vi "Query Protection Status.vi"(8 "error in (no error)":errorcluster, 10 "Channel (1)":string="1", 11 "VISA resource name":refnum<visa-resource-name>) -> (0 "error out":errorcluster, 1 "OCP Tripped":bool[](array[boolean]), 2 "OVP Tripped":bool[](array[boolean]), 3 "VISA resource name out":refnum<visa-resource-name>)   [LabVIEW 2020, in "Keysight E36300 Series.lvlib"]
doc: "Returns Overvoltage Protection (OVP) and Overcurrent Protection (OCP) status for a desired channel."
uses:
  Keysight E36300 Series.lvlib
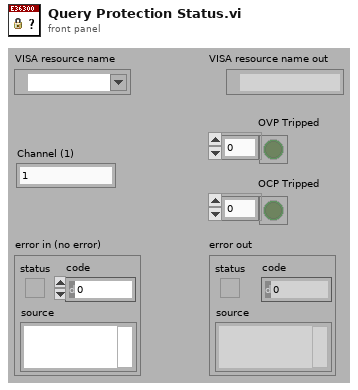
[diagram p1: front panel]
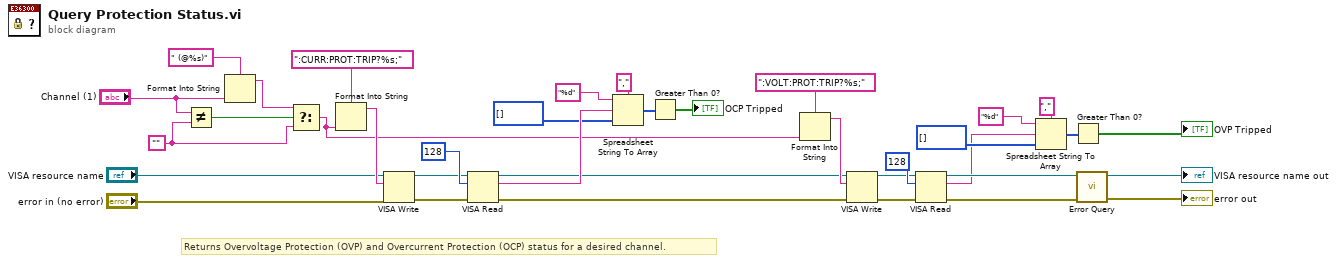
[diagram p0: block diagram]
diagram:
  w1 = ""
  # "Returns Overvoltage Protection (OVP) and Overcurrent Protection (OCP) status for a desired channel."
  n1 = Not Equal?(x="Channel (1)", y=w1) -> (x != y?=w4:bool)
  n2 = Format Into String(format string=" (@%s)", "Channel (1)") -> (resulting string=w5:string)  [unwired: 2 in, 1 out]
  n3 = Select(t=w5, s=w4, f=w1) -> (s? t:f=w2:string)
  n4 = Format Into String(format string=":CURR:PROT:TRIP?%s;", w2) -> (resulting string=w33:string)  [unwired: 2 in, 1 out]
  n5 = VISA Write(VISA resource name="VISA resource name", write buffer=w33, error in (no error)="error in (no error)") -> (VISA resource name out=w31:refnum<visa-resource-name>, error out=w30:errorcluster)  [unwired: 1 out]
  n6 = VISA Read(VISA resource name=w31, byte count=u32 128, error in (no error)=w30) -> (VISA resource name out=w17:refnum<visa-resource-name>, read buffer=w26:string, error out=w16:errorcluster)  [unwired: 1 out]
  n7 = Spreadsheet String To Array(delimiter (Tab)=",", format string="%d", spreadsheet string=w26, array type (2D Dbl)=i32[] []) -> (array=w18:i32[])
  n8 = Greater Than 0?(x=w18) -> (x > 0?=→"OCP Tripped":bool[])
  n9 = Format Into String(format string=":VOLT:PROT:TRIP?%s;", w2) -> (resulting string=w23:string)  [unwired: 2 in, 1 out]
  n10 = VISA Write(VISA resource name=w17, write buffer=w23, error in (no error)=w16) -> (VISA resource name out=w21:refnum<visa-resource-name>, error out=w20:errorcluster)  [unwired: 1 out]
  n11 = VISA Read(VISA resource name=w21, byte count=u32 128, error in (no error)=w20) -> (VISA resource name out=w15:refnum<visa-resource-name>, read buffer=w7:string, error out=w14:errorcluster)  [unwired: 1 out]
  n12 = Spreadsheet String To Array(delimiter (Tab)=",", format string="%d", spreadsheet string=w7, array type (2D Dbl)=i32[] []) -> (array=w10:i32[])
  n13 = Greater Than 0?(x=w10) -> (x > 0?=→"OVP Tripped":bool[])
  n14 = call "Error Query.vi"("error in (no error)"=w14, "VISA resource name"=w15) -> ("error out"=→"error out":errorcluster, "VISA resource name out"=→"VISA resource name out":refnum<visa-resource-name>)  [unwired: 6 in, 2 out]
